vi "Build Command Message.vi"(8 "error in (no error)":errorcluster, 10 "Command":string, 11 "Hitronics in":refnum<class "Hitronics.lvclass">) -> (0 "error out":errorcluster, 3 "Hitronics out":refnum<class "Hitronics.lvclass">)   [LabVIEW 2018, in "Hitronics.lvlib" / "Hitronics.lvclass"]
uses:
  Hitronics.lvclass
panel:
  out "Command String":string
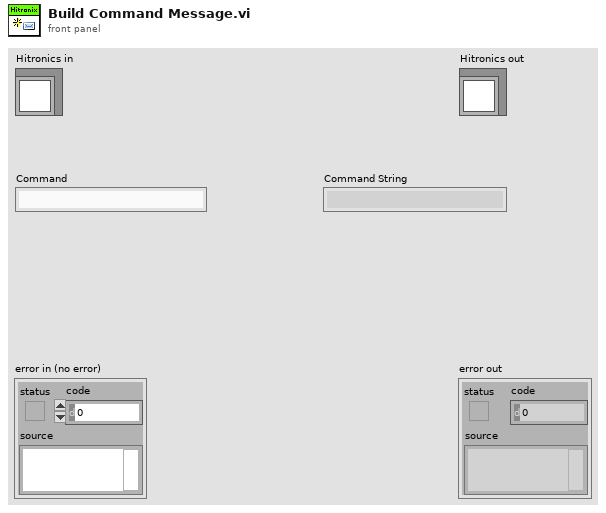
[diagram p1: front panel]
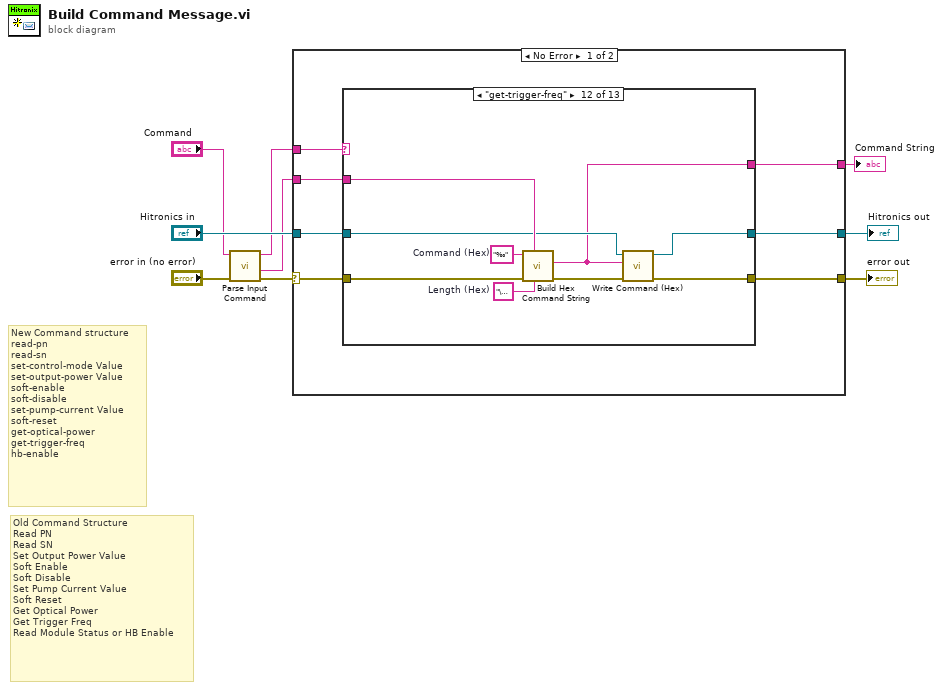
[diagram p0: block diagram]
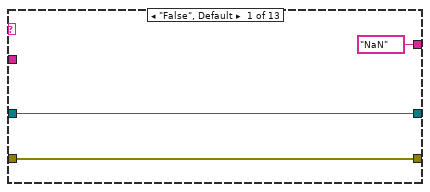
[diagram p2: hidden frame]
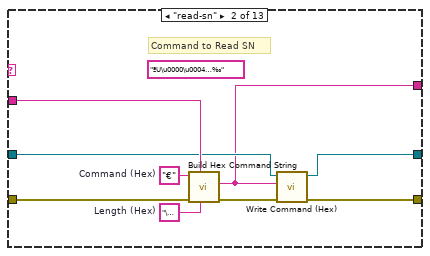
[diagram p3: hidden frame]
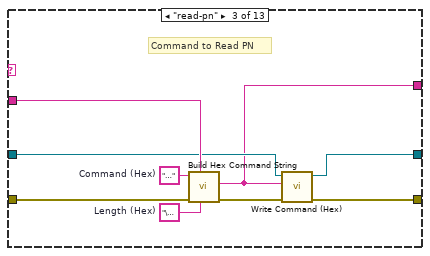
[diagram p4: hidden frame]
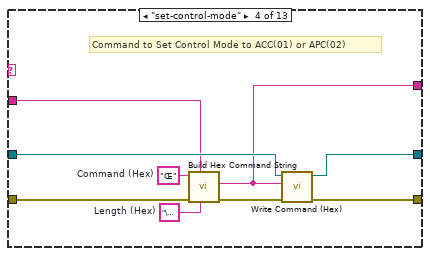
[diagram p5: hidden frame]
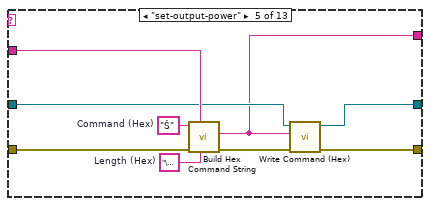
[diagram p6: hidden frame]
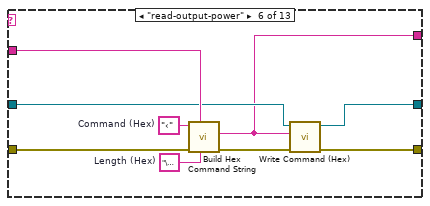
[diagram p7: hidden frame]
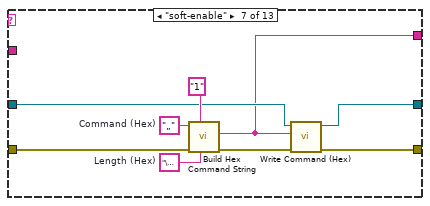
[diagram p8: hidden frame]
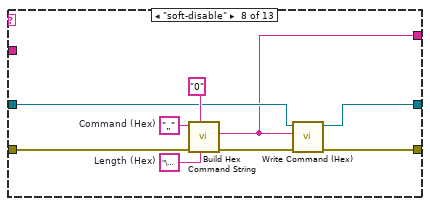
[diagram p9: hidden frame]
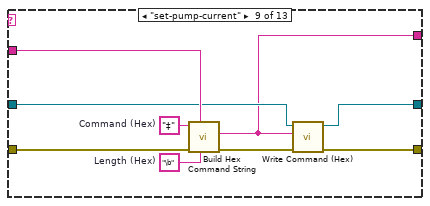
[diagram p10: hidden frame]
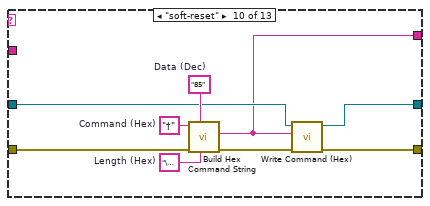
[diagram p11: hidden frame]
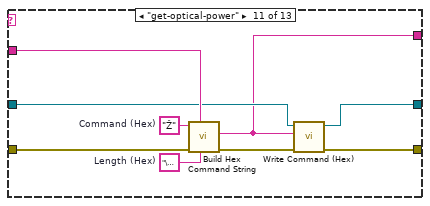
[diagram p12: hidden frame]
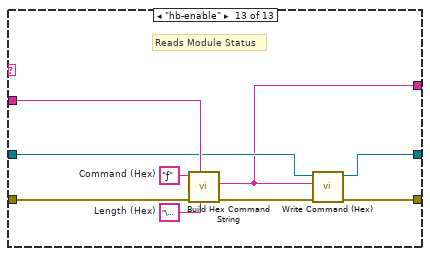
[diagram p13: hidden frame]
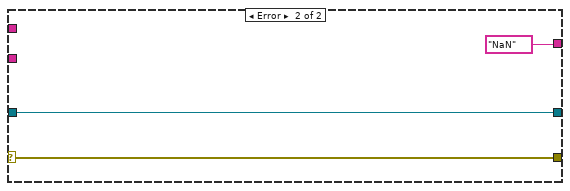
[diagram p14: hidden frame]
diagram:
  # "New Command structure\nread-pn \nread-sn\nset-control-mode Value\nset-output-power Value\nsoft-enable\nsoft-disable\nset-pump-current Value\nsoft-reset\nget-optical-power\nget-trigger-freq\nhb-enable"
  # "Old Command Structure\nRead PN \nRead SN\nSet Output Power Value\nSoft Enable\nSoft Disable\nSet Pump Current Value\nSoft Reset\nGet Optical Power\nGet Trigger Freq\nRead Module Status or HB Enable"
  n1 = call "Parse Input Command.vi"("Error In"="error in (no error)", "Command In"="Command") -> ("Error Out"=w2:errorcluster, "Value (Dec)"=w3:string, "Command Only"=w4:string)  [unwired: 7 in]
  n2 = case shown="No Error" w2 {
    selector: w2 -> [w14 w130]
    tunnel: [w12 w130] -> w9
    tunnel: [w13 w129] -> w7
    tunnel: "Hitronics in" -> [w15 w129]
    tunnel: w4 -> [w16 _]
    tunnel: w3 -> [w11 _]
    tunnel: [w10 "NaN" ("Command String")] -> w1
    frame No Error {
      n3 = case shown="\"get-trigger-freq\"" w16 {
        tunnel: w15 -> [w19 w23 w33 w43 w49 w58 w68 w76 w85 w94 w103 w112 w122]
        tunnel: w14 -> [w18 w28 w37 w46 w55 w64 w73 w82 w91 w100 w109 w118 w127]
        tunnel: [w19 w22 w30 w40 w48 w57 w67 w75 w84 w93 w102 w111 w121] -> w13
        tunnel: [w18 w21 w31 w41 w50 w59 w66 w77 w86 w95 w104 w113 w120] -> w12
        tunnel: w11 -> [_ w25 w34 w39 w52 w61 _ _ w88 _ w106 w115 w124]
        tunnel: ["NaN" ("Command String") w20 w29 w38 w47 w56 w65 w74 w83 w92 w101 w110 w119] -> w10
        frame "False", Default {
        }
        frame "read-sn" {
          w26 = "\u0004"  # Length (Hex)
          w27 = "€"  # Command (Hex)
          (unwired) "ªU\u0000\u0004…‰" ("Command")
          # "Command to Read SN"
          n4 = call "Build Hex Command String.vi"("Length"=w26, "Data (Dec)"=w25, "Error In"=w28, "Command (Hex)"=w27) -> ("Error Out"=w24:errorcluster, "Command String"=w20:string)  [unwired: 6 in]
          n5 = call-dynamic "Write Command (Hex).vi"("error in (no error)"=w24, "Command (Hex)"=w20, "Hitronics in"=w23) -> ("error out"=w21:errorcluster, "Hitronics out"=w22:refnum<class "Hitronics.lvclass">)  [unwired: 7 in]
        }
        frame "read-pn" {
          w35 = "\u0004"  # Length (Hex)
          w36 = "…"  # Command (Hex)
          # "Command to Read PN"
          n6 = call "Build Hex Command String.vi"("Length"=w35, "Data (Dec)"=w34, "Error In"=w37, "Command (Hex)"=w36) -> ("Error Out"=w32:errorcluster, "Command String"=w29:string)  [unwired: 6 in]
          n7 = call-dynamic "Write Command (Hex).vi"("error in (no error)"=w32, "Command (Hex)"=w29, "Hitronics in"=w33) -> ("error out"=w31:errorcluster, "Hitronics out"=w30:refnum<class "Hitronics.lvclass">)  [unwired: 7 in]
        }
        frame "set-control-mode" {
          w44 = "\u0006"  # Length (Hex)
          w45 = "Œ"  # Command (Hex)
          # "Command to Set Control Mode to ACC(01) or APC(02)"
          n8 = call "Build Hex Command String.vi"("Length"=w44, "Data (Dec)"=w39, "Error In"=w46, "Command (Hex)"=w45) -> ("Error Out"=w42:errorcluster, "Command String"=w38:string)  [unwired: 6 in]
          n9 = call-dynamic "Write Command (Hex).vi"("error in (no error)"=w42, "Command (Hex)"=w38, "Hitronics in"=w43) -> ("error out"=w41:errorcluster, "Hitronics out"=w40:refnum<class "Hitronics.lvclass">)  [unwired: 7 in]
        }
        frame "set-output-power" {
          w53 = "\u0006"  # Length (Hex)
          w54 = "Š"  # Command (Hex)
          n10 = call "Build Hex Command String.vi"("Length"=w53, "Data (Dec)"=w52, "Error In"=w55, "Command (Hex)"=w54) -> ("Error Out"=w51:errorcluster, "Command String"=w47:string)  [unwired: 6 in]
          n11 = call-dynamic "Write Command (Hex).vi"("error in (no error)"=w51, "Command (Hex)"=w47, "Hitronics in"=w49) -> ("error out"=w50:errorcluster, "Hitronics out"=w48:refnum<class "Hitronics.lvclass">)  [unwired: 7 in]
        }
        frame "read-output-power" {
          w62 = "\u0004"  # Length (Hex)
          w63 = "‹"  # Command (Hex)
          n12 = call "Build Hex Command String.vi"("Length"=w62, "Data (Dec)"=w61, "Error In"=w64, "Command (Hex)"=w63) -> ("Error Out"=w60:errorcluster, "Command String"=w56:string)  [unwired: 6 in]
          n13 = call-dynamic "Write Command (Hex).vi"("error in (no error)"=w60, "Command (Hex)"=w56, "Hitronics in"=w58) -> ("error out"=w59:errorcluster, "Hitronics out"=w57:refnum<class "Hitronics.lvclass">)  [unwired: 7 in]
        }
        frame "soft-enable" {
          w71 = "\u0005"  # Length (Hex)
          w72 = "„"  # Command (Hex)
          n14 = call "Build Hex Command String.vi"("Length"=w71, "Data (Dec)"="1", "Error In"=w73, "Command (Hex)"=w72) -> ("Error Out"=w69:errorcluster, "Command String"=w65:string)  [unwired: 6 in]
          n15 = call-dynamic "Write Command (Hex).vi"("error in (no error)"=w69, "Command (Hex)"=w65, "Hitronics in"=w68) -> ("error out"=w66:errorcluster, "Hitronics out"=w67:refnum<class "Hitronics.lvclass">)  [unwired: 7 in]
        }
        frame "soft-disable" {
          w80 = "\u0005"  # Length (Hex)
          w81 = "„"  # Command (Hex)
          n16 = call "Build Hex Command String.vi"("Length"=w80, "Data (Dec)"="0", "Error In"=w82, "Command (Hex)"=w81) -> ("Error Out"=w78:errorcluster, "Command String"=w74:string)  [unwired: 6 in]
          n17 = call-dynamic "Write Command (Hex).vi"("error in (no error)"=w78, "Command (Hex)"=w74, "Hitronics in"=w76) -> ("error out"=w77:errorcluster, "Hitronics out"=w75:refnum<class "Hitronics.lvclass">)  [unwired: 7 in]
        }
        frame "set-pump-current" {
          w89 = "\b"  # Length (Hex)
          w90 = "‡"  # Command (Hex)
          n18 = call "Build Hex Command String.vi"("Length"=w89, "Data (Dec)"=w88, "Error In"=w91, "Command (Hex)"=w90) -> ("Error Out"=w87:errorcluster, "Command String"=w83:string)  [unwired: 6 in]
          n19 = call-dynamic "Write Command (Hex).vi"("error in (no error)"=w87, "Command (Hex)"=w83, "Hitronics in"=w85) -> ("error out"=w86:errorcluster, "Hitronics out"=w84:refnum<class "Hitronics.lvclass">)  [unwired: 7 in]
        }
        frame "soft-reset" {
          w97 = "85"  # Data (Dec)
          w98 = "\u0005"  # Length (Hex)
          w99 = "†"  # Command (Hex)
          n20 = call "Build Hex Command String.vi"("Length"=w98, "Data (Dec)"=w97, "Error In"=w100, "Command (Hex)"=w99) -> ("Error Out"=w96:errorcluster, "Command String"=w92:string)  [unwired: 6 in]
          n21 = call-dynamic "Write Command (Hex).vi"("error in (no error)"=w96, "Command (Hex)"=w92, "Hitronics in"=w94) -> ("error out"=w95:errorcluster, "Hitronics out"=w93:refnum<class "Hitronics.lvclass">)  [unwired: 7 in]
        }
        frame "get-optical-power" {
          w107 = "\u0004"  # Length (Hex)
          w108 = "Ž"  # Command (Hex)
          n22 = call "Build Hex Command String.vi"("Length"=w107, "Data (Dec)"=w106, "Error In"=w109, "Command (Hex)"=w108) -> ("Error Out"=w105:errorcluster, "Command String"=w101:string)  [unwired: 6 in]
          n23 = call-dynamic "Write Command (Hex).vi"("error in (no error)"=w105, "Command (Hex)"=w101, "Hitronics in"=w103) -> ("error out"=w104:errorcluster, "Hitronics out"=w102:refnum<class "Hitronics.lvclass">)  [unwired: 7 in]
        }
        frame "get-trigger-freq" {
          w116 = "\u0004"  # Length (Hex)
          w117 = "‰"  # Command (Hex)
          n24 = call "Build Hex Command String.vi"("Length"=w116, "Data (Dec)"=w115, "Error In"=w118, "Command (Hex)"=w117) -> ("Error Out"=w114:errorcluster, "Command String"=w110:string)  [unwired: 6 in]
          n25 = call-dynamic "Write Command (Hex).vi"("error in (no error)"=w114, "Command (Hex)"=w110, "Hitronics in"=w112) -> ("error out"=w113:errorcluster, "Hitronics out"=w111:refnum<class "Hitronics.lvclass">)  [unwired: 7 in]
        }
        frame "hb-enable" {
          w125 = "\u0004"  # Length (Hex)
          w126 = "ƒ"  # Command (Hex)
          # "Reads Module Status"
          n26 = call "Build Hex Command String.vi"("Length"=w125, "Data (Dec)"=w124, "Error In"=w127, "Command (Hex)"=w126) -> ("Error Out"=w123:errorcluster, "Command String"=w119:string)  [unwired: 6 in]
          n27 = call-dynamic "Write Command (Hex).vi"("error in (no error)"=w123, "Command (Hex)"=w119, "Hitronics in"=w122) -> ("error out"=w120:errorcluster, "Hitronics out"=w121:refnum<class "Hitronics.lvclass">)  [unwired: 7 in]
        }
      }
    }
    frame Error {
    }
  }
  "error out" <- w9
  "Hitronics out" <- w7
  "Command String" <- w1
